vi "N4_201_check_mode.vi"(4 "Driver Name":T10, 5 "Delay befor,s":T6=2.0, 6 "Error Code":T9, 7 "InputParam":T7, 8 "error in":T8, 11 "DriverConnect in":T1={"InterfaceType"=enum."VISA", "OpenedSession"="", "InterfaceSettings"={"Interface"=enum."RS232", "EOS 4 read"=enum."LF (\\n)", "EOS 4 write"=enum."LF (\\n)", "TMO, ms"=10000, "Sett"=variant(cluster{"Baud Rate":u32, "Data Bits":u16, "Parity":u16, "Stop Bits":u16, "Flow Control":u16, "Eho":bool} {"Baud Rate"=75, "Data Bits"=0, "Parity"=0, "Stop Bits"=0, "Flow Control"=0, "Eho"=FALSE})}}) -> (0 "error out":T8, 3 "DriverConnect out":T1={"InterfaceType"=enum."VISA", "OpenedSession"="", "InterfaceSettings"={"Interface"=enum."RS232", "EOS 4 read"=enum."LF (\\n)", "EOS 4 write"=enum."LF (\\n)", "TMO, ms"=10000, "Sett"=variant(cluster{"Baud Rate":u32, "Data Bits":u16, "Parity":u16, "Stop Bits":u16, "Flow Control":u16, "Eho":bool} {"Baud Rate"=75, "Data Bits"=0, "Parity"=0, "Stop Bits"=0, "Flow Control"=0, "Eho"=FALSE})}})   [LabVIEW 2018]
uses:
  MOKO_LabViewLibrary/MokoLowLevel/MokoLowLovelControl/MLLC_DriverName.ctl
  MOKO_LabViewLibrary/MokoLowLevel/MokoLowLovelControl/MLLC_ErrorCode.ctl
  MOKO_LabViewLibrary/MokoLowLevel/MokoLowLovelControl/MLLC_Error.ctl
  MOKO_LabViewLibrary/MokoLowLevel/MokoLowLovelControl/MLLC_Command.ctl
  MOKO_LabViewLibrary/MokoLowLevel/MokoLowLovelControl/MLLC_Delay.ctl
  MOKO_LabViewLibrary/MokoLowLevel/MokoLowLovelControl/MLLC_ConnectCluster.ctl
  MOKO_LabViewLibrary/MokoLowLevel/MokoLowLovelControl/MLLC_InterfaceType.ctl
  MOKO_LabViewLibrary/MokoLowLevel/MokoLowLovelControl/MLLC_OpenedSession.ctl
  MOKO_LabViewLibrary/MokoLowLevel/MokoLowLovelControl/MLLC_InterfaceSettings.ctl
  MOKO_LabViewLibrary/MokoLowLevel/MokoLowLovelControl/MLLC_InterfaceKind.ctl
panel:
  in  "InputMode":T7
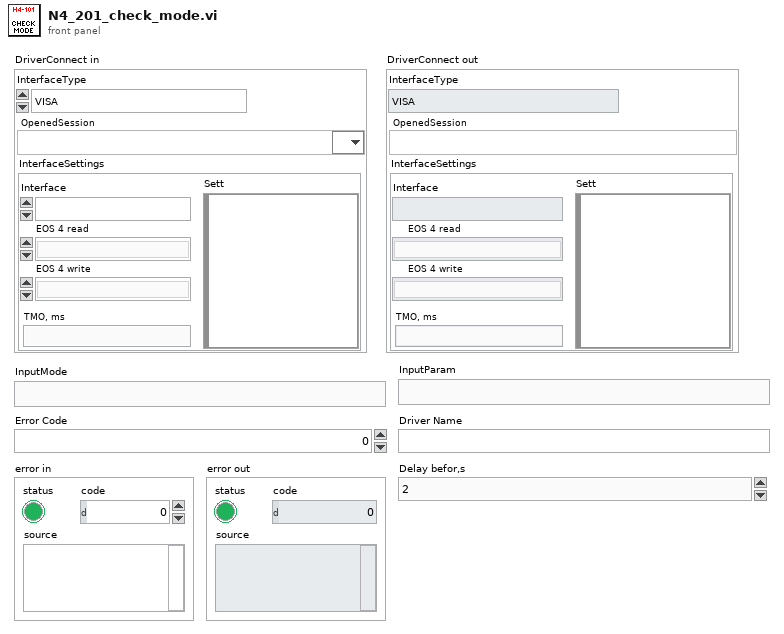
[diagram p1: front panel]
types:
  T1 = typedef "MLLC_ConnectCluster.ctl" = cluster{"InterfaceType":T2, "OpenedSession":T3, "InterfaceSettings":T4}
  T2 = typedef "MLLC_InterfaceType.ctl" = enum16{"VISA", "Prologix USB-GPIB"}
  T3 = typedef "MLLC_OpenedSession.ctl" = refnum<visa-resource-name>
  T4 = typedef "MLLC_InterfaceSettings.ctl" = cluster{"Interface":T5, "EOS 4 read":enum16{"Default (=EOS 4 write)", "CR (\\r)", "LF (\\n)", "None"}, "EOS 4 write":enum16{"CR+LF (\\r\\n)", "CR (\\r)", "LF (\\n)", "None"}, "TMO, ms":i32, "Sett":variant}
  T5 = typedef "MLLC_InterfaceKind.ctl" = enum16{"RS232", "GPIB", "USB", "Ethernet", "another"}
  T6 = typedef "MLLC_Delay.ctl" = dbl
  T7 = typedef "MLLC_Command.ctl" = string
  T8 = typedef "MLLC_Error.ctl" = errorcluster
  T9 = typedef "MLLC_ErrorCode.ctl" = u32
  T10 = typedef "MLLC_DriverName.ctl" = string
  T11 = enum16{"Нет симуляции", "В ручную", "Игнорировать"}
  T12 = typedef "MLLC_Response.ctl" = string
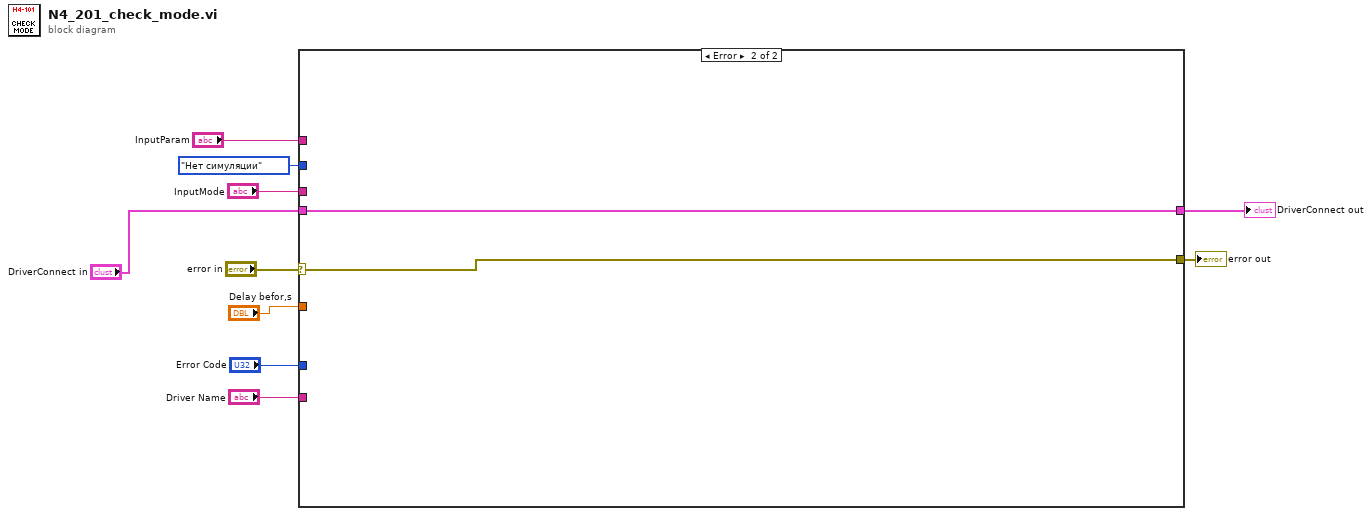
[diagram p0: block diagram]
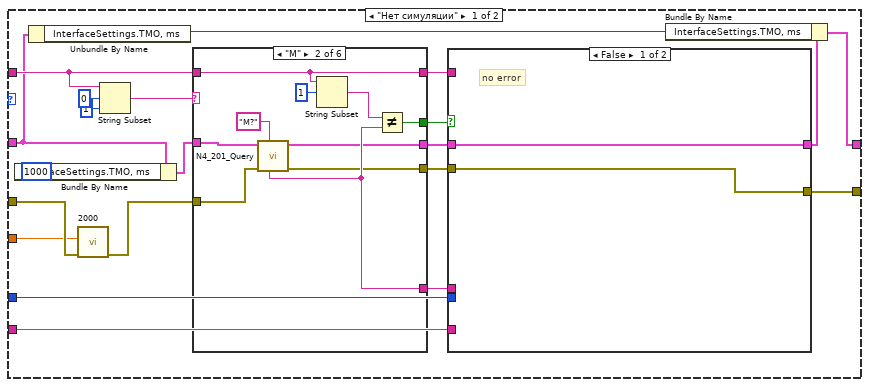
[diagram p3: hidden frame]
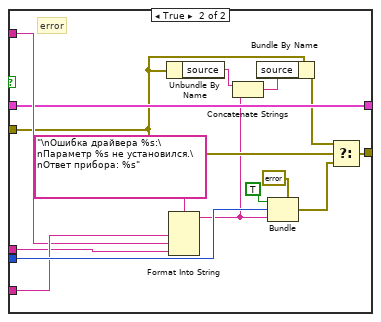
[diagram p4: hidden frame]
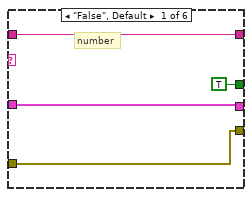
[diagram p5: hidden frame]
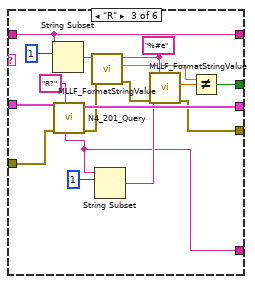
[diagram p6: hidden frame]
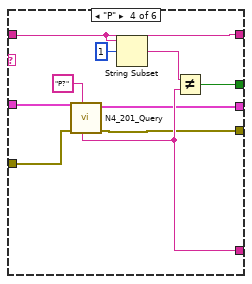
[diagram p7: hidden frame]
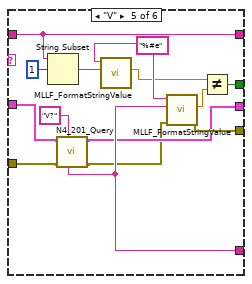
[diagram p8: hidden frame]
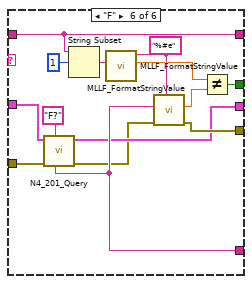
[diagram p9: hidden frame]
diagram:
  n1 = case shown="Error" "error in" {
    selector: "error in" -> [w18 w129]
    tunnel: "DriverConnect in" -> [w19 w130]
    tunnel: "Error Code" -> [w14 _]
    tunnel: "Driver Name" -> [w13 _]
    tunnel: [w17 w130] -> w1
    tunnel: [w16 w129] -> w7
    tunnel: "InputMode" -> [_ _]
    tunnel: "InputParam" -> [w15 _]
    tunnel: T11."Нет симуляции" ("Simmulation") -> [w12 _]
    tunnel: "Delay befor,s" -> [w11 _]
    frame No Error {
      n2 = case shown="\"В ручную\", Default" w12 {
        tunnel: w19 -> [w23 w127]
        tunnel: w18 -> [w28 w128]
        tunnel: [w20 w127] -> w17
        tunnel: [w38 w128] -> w16
        tunnel: w15 -> [w33 _]
        tunnel: w14 -> [w31 _]
        tunnel: w13 -> [w30 _]
        tunnel: w11 -> [w26 _]
        frame "Нет симуляции" {
          n3 = Bundle By Name(cluster=w23, "InterfaceSettings.TMO, ms"=1000 ("TMO, ms")) -> (w22:T1)
          n4 = Unbundle By Name(w23) -> ("InterfaceSettings.TMO, ms"=w24:i32)
          n5 = call "2000"("error in (no error)"=w28, "Delay Time (s)"=w26) -> ("error out"=w27:errorcluster)  [unwired: 9 in]
          n6 = String Subset(string=w33, offset (0)=0, length (rest)=1 ("length (rest)")) -> (substring=w35:T7)
          n7 = case shown="\"M\"" w35 {
            tunnel: w22 -> [w59 w70 w87 w97 w101 w125]
            tunnel: w27 -> [w58 w69 w86 w96 w103 w124]
            tunnel: [w59 w63 w84 w89 w100 w114] -> w39
            tunnel: [w58 w62 w78 w90 w105 w116] -> w37
            tunnel: [TRUE w67 w85 w95 w112 w123] -> w40
            tunnel: w33 -> [w60 w65 w76 w92 w106 w117]
            tunnel: [w60 w65 w76 w92 w106 w117] -> w32
            tunnel: [_ w64 w72 w91 w104 w115] -> w29
            frame "False", Default {
              # "number"
            }
            frame "M" {
              n8 = call "N4_201_Query.vi"("Command"="M?" ("Error Query"), "error in"=w69, "DriverConnect in"=w70) -> ("error out"=w62:T8, "DriverConnect out"=w63:T1, "Response"=w64:T12)  [unwired: 6 in]
              n9 = String Subset(string=w65, offset (0)=1) -> (substring=w66:T7)  [unwired: 1 in]
              n10 = Not Equal?(x=w66, y=w64) -> (x != y?=w67:bool)
            }
            frame "R" {
              w83 = "%#e" ("format string")
              n11 = String Subset(string=w76, offset (0)=1) -> (substring=w75:T7)  [unwired: 1 in]
              n12 = call "N4_201_Query.vi"("Command"="R?" ("Error Query"), "error in"=w86, "DriverConnect in"=w87) -> ("error out"=w80:T8, "DriverConnect out"=w84:T1, "Response"=w72:T12)  [unwired: 6 in]
              n13 = call "MLLF_FormatStringValue.vi"("error in"=w80, "String Value"=w75, "Format"=w83) -> ("error out"=w79:T8, "number"=w81:dbl)  [unwired: 6 in, 1 out]
              n14 = String Subset(string=w72, offset (0)=1) -> (substring=w73:T12)  [unwired: 1 in]
              n15 = call "MLLF_FormatStringValue.vi"("error in"=w79, "String Value"=w73, "Format"=w83) -> ("error out"=w78:T8, "number"=w82:dbl)  [unwired: 6 in, 1 out]
              n16 = Not Equal?(x=w81, y=w82) -> (x != y?=w85:bool)
            }
            frame "P" {
              n17 = call "N4_201_Query.vi"("Command"="P?" ("Error Query"), "error in"=w96, "DriverConnect in"=w97) -> ("error out"=w90:T8, "DriverConnect out"=w89:T1, "Response"=w91:T12)  [unwired: 6 in]
              n18 = String Subset(string=w92, offset (0)=1) -> (substring=w93:T7)  [unwired: 1 in]
              n19 = Not Equal?(x=w93, y=w91) -> (x != y?=w95:bool)
            }
            frame "V" {
              w109 = "%#e" ("format string")
              n20 = String Subset(string=w106, offset (0)=1) -> (substring=w110:T7)  [unwired: 1 in]
              n21 = call "N4_201_Query.vi"("Command"="V?" ("Error Query"), "error in"=w103, "DriverConnect in"=w101) -> ("error out"=w99:T8, "DriverConnect out"=w100:T1, "Response"=w104:T12)  [unwired: 6 in]
              n22 = call "MLLF_FormatStringValue.vi"("String Value"=w110, "Format"=w109) -> ("number"=w108:dbl)  [unwired: 7 in, 2 out]
              n23 = call "MLLF_FormatStringValue.vi"("error in"=w99, "String Value"=w104, "Format"=w109) -> ("error out"=w105:T8, "number"=w107:dbl)  [unwired: 6 in, 1 out]
              n24 = Not Equal?(x=w108, y=w107) -> (x != y?=w112:bool)
            }
            frame "F" {
              w120 = "%#e" ("format string")
              n25 = call "N4_201_Query.vi"("Command"="F?" ("Error Query"), "error in"=w124, "DriverConnect in"=w125) -> ("error out"=w113:T8, "DriverConnect out"=w114:T1, "Response"=w115:T12)  [unwired: 6 in]
              n26 = String Subset(string=w117, offset (0)=1) -> (substring=w121:T7)  [unwired: 1 in]
              n27 = call "MLLF_FormatStringValue.vi"("String Value"=w121, "Format"=w120) -> ("number"=w119:dbl)  [unwired: 7 in, 2 out]
              n28 = call "MLLF_FormatStringValue.vi"("error in"=w113, "String Value"=w115, "Format"=w120) -> ("error out"=w116:T8, "number"=w118:dbl)  [unwired: 6 in, 1 out]
              n29 = Not Equal?(x=w119, y=w118) -> (x != y?=w123:bool)
            }
          }
          n30 = case shown="False" w40 {
            tunnel: w39 -> [w42 w51]
            tunnel: [w42 w51] -> w21
            tunnel: [w41 w43] -> w38
            tunnel: w37 -> [w41 w49]
            tunnel: w32 -> [_ w52]
            tunnel: w31 -> [_ w54]
            tunnel: w30 -> [_ w53]
            tunnel: w29 -> [_ w50]
            frame False {
              # "no error"
            }
            frame True {
              # "error"
              n31 = Unbundle By Name(w49) -> ("source"=w48:string)
              n32 = Format Into String(format string="\nОшибка драйвера %s:\nПараметр %s не установился.\nОтвет прибора: %s", w53, w52, w50) -> (resulting string=w46:string)  [unwired: 2 in, 1 out]
              n33 = Concatenate Strings(w48, w46) -> (w47:string)
              n34 = Bundle By Name(cluster=w49, "source"=w47) -> (w45:T8)
              n35 = Bundle(cluster=errorcluster {"status"=FALSE, "code"=0, "source"=""} ("error out"), "status"=TRUE ("Status"), "code"=w54, "source"=w46) -> (w44:errorcluster)
              n36 = Select(t=w45, s=w49, f=w44) -> (s? t:f=w43:T8)
            }
          }
          n37 = Bundle By Name(cluster=w21, "InterfaceSettings.TMO, ms"=w24) -> (w20:T1)
        }
        frame "В ручную", Default {
        }
      }
    }
    frame Error {
    }
  }
  "error out" <- w7
  "DriverConnect out" <- w1
